vi "RTShutter.vi"(8 "error in (no error)":errorcluster) -> (0 "error out":errorcluster)   [LabVIEW 2016]
uses:
  Classes/Shutter/Container/Container.lvclass
  <vilib>/Platform/TimedLoop/XDataNode/timing_clust.ctl
  <vilib>/Platform/TimedLoop/XDataNode/nitl_modes.ctl
  <vilib>/Platform/TimedLoop/XDataNode/wakeup.ctl
  Controls/Operational Modes.ctl
  Controls/Shutters.ctl
  Controls/Shutter Data.ctl
  Controls/Shutter States.ctl
  <vilib>/Platform/TimedLoop/XDataNode/loadnilvce.vi
  <vilib>/platform/TimedLoop/XDataNode/XDataNode.xnode
  <vilib>/Platform/TimedLoop/XDataNode/XDNodeRunTimeDep.lvlib
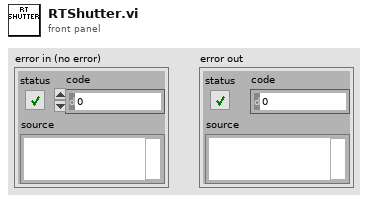
[diagram p1: front panel]
types:
  T1 = typedef "XDNodeRunTimeDep.lvlib/timing_clust.ctl" = cluster{"Expected End [f-1]":u64, "Actual End [f-1]":u64, "Finished Late? [f-1]":bool, "Expected End [i-1]":u64, "Actual End [i-1]":u64, "Finished Late? [i-1]":bool, "Expected Start [i]":u64, "Actual Start [i]":u64, "Expected Start [f]":u64, "Actual Start [f]":u64, "Source Name":string, "Structure Name":string, "Period":i64, "Deadline":i64, "Offset":i64, "Start":i64, "Priority":i32, "Timeout":i32, "Mode":T2, "Wakeup Reason":T3, "Error":errorcluster, "Source Type":string, "Secondary Source Type":string, "Global End Time":u64, "Global Start Time":u64, "Frame Duration":u64, "Iteration Duration":u64, "Assigned CPU":i32, "I/O Scan Engine Mode":u32}
  T2 = typedef "XDNodeRunTimeDep.lvlib/nitl_modes.ctl" = enum32{"No Change", "Process missed periods, maintain original phase", "Discard missed periods, maintain original phase", "Process missed periods, ignore original phase", "Discard missed periods, ignore original phase"}
  T3 = typedef "XDNodeRunTimeDep.lvlib/wakeup.ctl" = enum32{"Normal", "Aborted", "Asynchronous wakeup", "Timing source error", "Timed loop error", "Timeout"}
  T4 = typedef "Operational Modes.ctl" = enum16{"Sci", "Sci-LFC", "Solar", "Solar-LFC", "LFC", "LFC-Sim", "LFC-Both", "ThAr", "ThAr-LFC", "Flat", "ExtFlat", "ExtFlat-Sim", "ExtFlat-Both", "Qtz", "ExtQtz", "ExtQtz-Sim", "ExtQtz-Both", "Dark", "Manual", "Off"}
  T5 = typedef "Shutters.ctl" = cluster{"Science":T6, "LFCSim":T6, "ExtendFlat":T6, "SimFlat":T6, "Solar":T6}
  T6 = typedef "Shutter Data.ctl" = cluster{"Status":bool, "State":T7, "Time Stamps":cluster{"Open":timestamp, "Close":timestamp}, "Exposure Time":dbl}
  T7 = typedef "Shutter States.ctl" = enum16{"Open", "Close", "Wait", "Off", "Arm", "Idle"}
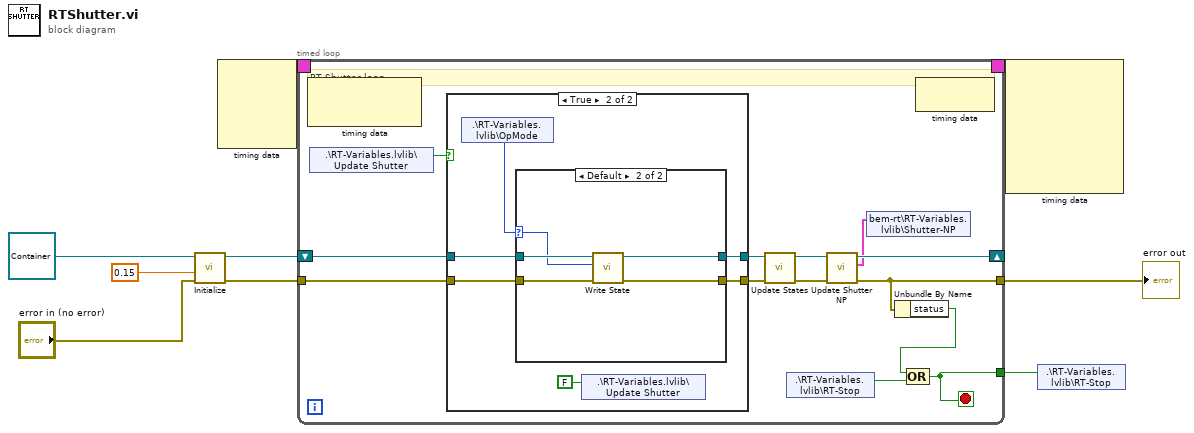
[diagram p0: block diagram]
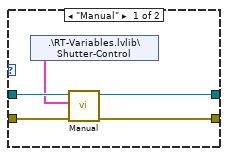
[diagram p3: hidden frame]
diagram:
  n1 = call-dynamic "Initialize.vi"("error in (no error)"="error in (no error)", "Power time"=0.15, "Container in"=refnum<class "Container.lvclass"> refnum ("Container.lvclass")) -> ("error out"=w7:errorcluster, "Container out"=w6:refnum<class "Container.lvclass">)  [unwired: 7 in]
  n2 = node-c288() -> (w2:T1)  [unwired: 4 in]
  n3 = timed-loop {
    tunnel: [w21] -> w4
    shift-right: [w16] -> _
    shift-left: w6 -> [w19]
    tunnel: w7 -> [w18]
    tunnel: [w15] -> w3
    timing: w2 -> [_]
    timing-out: [_] -> w1
    stop <- w21 stop-if-true
    # "RT Shutter loop"
    n4 = node-c288() -> ()  [unwired: 1 in, 2 out]
    n5 = shared-variable ".\\RT-Variables.lvlib\\Update Shutter"() -> (w20:bool)  [unwired: 1 in, 1 out]
    n6 = case shown="True" w20 {
      tunnel: w19 -> [w25 w32]
      tunnel: [w25 w31] -> w14
      tunnel: w18 -> [w26 w30]
      tunnel: [w26 w29] -> w13
      frame False {
      }
      frame True {
        n7 = shared-variable ".\\RT-Variables.lvlib\\OpMode"() -> (w27:T4)  [unwired: 1 in, 1 out]
        n8 = case shown="Default" w27 {
          selector: w27 -> [_ w38]
          tunnel: w32 -> [w35 w42]
          tunnel: [w37 w41] -> w31
          tunnel: w30 -> [w33 w40]
          tunnel: [w36 w39] -> w29
          frame "Manual" {
            n9 = shared-variable ".\\RT-Variables.lvlib\\Shutter-Control"() -> (w34:T5)  [unwired: 1 in, 1 out]
            n10 = call-dynamic "Manual.vi"("error in (no error)"=w33, "Shutters"=w34, "Container in"=w35) -> ("error out"=w36:errorcluster, "Container out"=w37:refnum<class "Container.lvclass">)  [unwired: 7 in]
          }
          frame Default {
            n11 = call-dynamic "Write State.vi"("error in (no error)"=w40, "OpMode"=w38, "Container in"=w42) -> ("error out"=w39:errorcluster, "Container out"=w41:refnum<class "Container.lvclass">)  [unwired: 7 in]
          }
        }
        n12 = shared-variable ".\\RT-Variables.lvlib\\Update Shutter"(FALSE ("Update?")) -> ()  [unwired: 1 in, 1 out]
      }
    }
    n13 = call-dynamic "Update States.vi"("error in (no error)"=w13, "Container in"=w14) -> ("error out"=w12:errorcluster, "Container out"=w11:refnum<class "Container.lvclass">)  [unwired: 8 in]
    n14 = shared-variable ".\\RT-Variables.lvlib\\RT-Stop"() -> (w22:bool)  [unwired: 1 in, 1 out]
    n15 = call "Update Shutter NP.vi"("error in (no error)"=w12, "Container in"=w11) -> ("error out"=w15:errorcluster, "Shutter-NP out"=w10:T5, "Container out"=w16:refnum<class "Container.lvclass">)  [unwired: 7 in]
    n16 = shared-variable "bem-rt\\RT-Variables.lvlib\\Shutter-NP"(w10) -> ()  [unwired: 1 in, 1 out]
    n17 = Unbundle By Name(w15) -> ("status"=w17:bool)
    n18 = Compound Arithmetic op=OR(w17, w22) -> (w21:bool)
    n19 = node-c288() -> ()  [unwired: 1 in, 1 out]
  }
  "error out" <- w3
  n20 = node-c288(w1) -> ()  [unwired: 7 out]
  n21 = shared-variable ".\\RT-Variables.lvlib\\RT-Stop"(w4) -> ()  [unwired: 1 in, 1 out]
